vi "Read Resource.vi"(8 "error in (no error)":errorcluster, 11 "EXFO in":refnum<class "EXFO.lvclass">) -> (0 "error out":errorcluster, 2 "Resource":refnum<visa-resource-name>, 3 "EXFO out":refnum<class "EXFO.lvclass">)   [LabVIEW 2018, in "EXFO.lvlib" / "EXFO.lvclass"]
doc: "This is a parent VI, used to provide resource information to the children classes. It can be accessed through the property node. \n\n\nAuthor: Ron Dexter\nCompany: Luminar\nModified: 5/20/2018"
uses:
  EXFO.lvclass
  EXFO.lvclass/EXFO.ctl
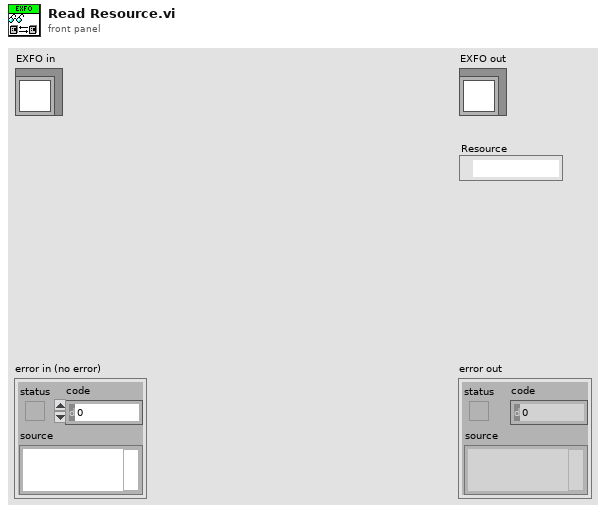
[diagram p1: front panel]
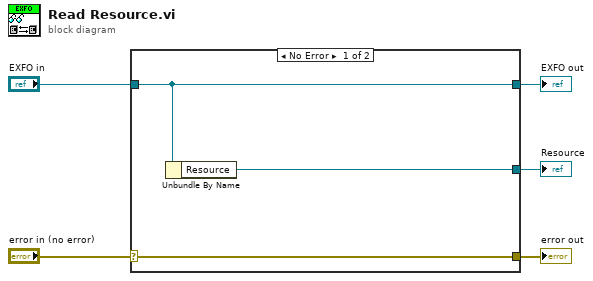
[diagram p0: block diagram]
diagram:
  n1 = case shown="No Error" "error in (no error)" {
    selector: "error in (no error)" -> [w8 w9]
    tunnel: [w8 w9] -> w4
    tunnel: [w7 w10] -> w2
    tunnel: "EXFO in" -> [w7 w10]
    tunnel: [w6 _] -> w1
    frame No Error {
      n2 = Unbundle By Name(w7) -> ("Resource"=w6:refnum<visa-resource-name>)
    }
    frame Error {
    }
  }
  "error out" <- w4
  "EXFO out" <- w2
  "Resource" <- w1
